vi "COP Transport Layer.vi"() -> ()   [LabVIEW 2011]
uses:
  Support Files/JUDP Read Queue Element.ctl
  Support Files/Address.ctl
  Support Files/JUDP Write Queue Element.ctl
  cRIO/Functional Global Variables/Actions for FG's.ctl
panel:
  out "UDP Write Loop":bool
  out "UDP Read Loop":bool
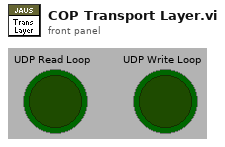
[diagram p1: front panel]
types:
  T1 = typedef "JUDP Write Queue Element.ctl" = cluster{"Encoded JAUS Message":string, "Destination ID":u32}
  T2 = typedef "JUDP Read Queue Element.ctl" = cluster{"Payload":string, "Sender ID":T3, "Command Code":u16}
  T3 = typedef "Address.ctl" = cluster{"Subsystem Id":u16, "Node Id":u8, "Component Id":u8}
  T4 = typedef "UDP Base.ctl" = cluster{"UDP Session":refnum<k16>, "UDP Socket Params":T5}
  T5 = typedef "UDP Socket Params.ctl" = cluster{"Local Port":u16, "Read Timeout":i32, "Write Timeout":i32}
  T6 = typedef "Actions for FG's.ctl" = enum16{"Read", "Write"}
  T7 = cluster{"QueryType":u8, "Type":u16, "COP Identification":string}
  T8 = typedef "UDP Network Location.ctl" = cluster{"IP Address":string, "Port":u16}
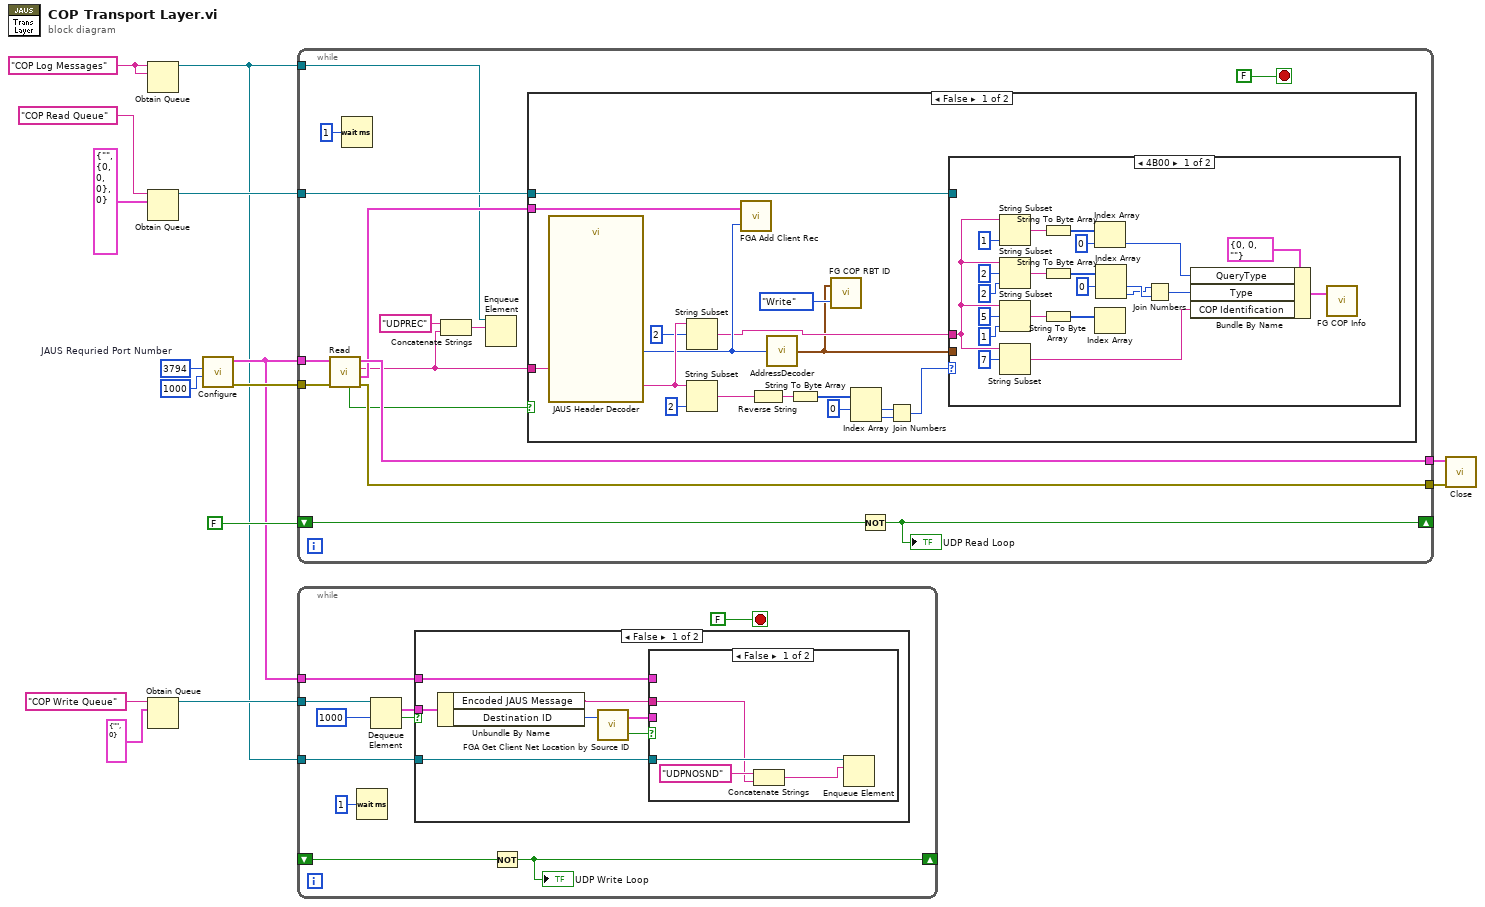
[diagram p0: block diagram]
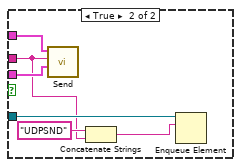
[diagram p2: hidden frame]
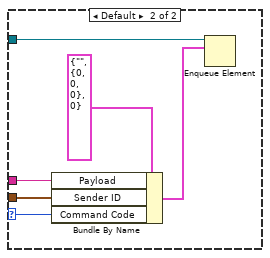
[diagram p4: hidden frame]
diagram:
  w2 = "COP Log Messages" ("name (unnamed)")
  w11 = u16 3794  # JAUS Requried Port Number
  n1 = Obtain Queue(name (unnamed)=w2, element data type=w2) -> (queue out=w1:refnum<queue>)  [unwired: 3 in, 2 out]
  n2 = Obtain Queue(name (unnamed)="COP Read Queue", element data type=T2 {"Payload"="", "Sender ID"={"Subsystem Id"=0, "Node Id"=0, "Component Id"=0}, "Command Code"=0} ("Receive FSM Queue Element")) -> (queue out=w13:refnum<queue>)  [unwired: 3 in, 2 out]
  n3 = Obtain Queue(name (unnamed)="COP Write Queue", element data type=T1 {"Encoded JAUS Message"="", "Destination ID"=0} ("Cluster")) -> (queue out=w6:refnum<queue>)  [unwired: 3 in, 2 out]
  n4 = call "Configure.vi"("Read Timeout"=1000, "Local Port"=w11) -> ("error out"=w12:errorcluster, "UDP Base out"=w3:T4)  [unwired: 8 in]
  n5 = while {
    tunnel: w13 -> [w30]
    tunnel: w3 -> [w28]
    tunnel: w12 -> [w29]
    tunnel: [w27] -> w9
    tunnel: [w26] -> w8
    shift-right: [w24] -> _
    shift-left: FALSE ("stop") -> [w25]
    tunnel: w1 -> [w19]
    stop <- FALSE stop-if-true
    n6 = call "Read.vi"("error in (no error)"=w29, "UDP Base in"=w28) -> ("error out"=w26:errorcluster, "Network Location"=w22:T8, "Receive Data"=w16:string, "UDP Base out"=w27:T4, "Timeout"=w23:bool)  [unwired: 4 in, 1 out]
    n7 = Wait (ms)(milliseconds to wait=u32 1) -> ()  [unwired: 1 out]
    n8 = Concatenate Strings("UDPREC" ("string"), w16) -> (w18:string)
    n9 = Enqueue Element(queue=w19, element=w18) -> ()  [unwired: 2 in, 3 out]
    n10 = case shown="False" w23 {
      tunnel: w30 -> [w36 _]
      tunnel: w16 -> [w38 _]
      tunnel: w22 -> [w37 _]
      frame False {
        n11 = call "JAUS Header Decoder.vi"("Encoded JAUS Message"=w38) -> ("Source ID (80-95)"=w35:u32, "Payload"=w40:string)  [unwired: 13 in, 12 out]
        n12 = String Subset(string=w40, offset (0)=2) -> (substring=w34:string)  [unwired: 1 in]
        n13 = String Subset(string=w40, length (rest)=2 ("length (rest)")) -> (substring=w41:string)  [unwired: 1 in]
        n14 = call "FGA Add Client Rec.vi"("ID"=w35, "Network Location"=w37) -> ()  [unwired: 1 in, 1 out]
        n15 = Reverse String(1:w41) -> (0:w43:string)
        n16 = call "AddressDecoder.vi"("Address"=w35) -> ("Address Cluster"=w31:T3)
        n17 = String To Byte Array(string=w43) -> (unsigned byte array=w47:u8[])
        n18 = call "FG COP RBT ID.vi"("FG Action (Read)"=Actions_for_FG's."Write", "RBT ID in"=w31) -> ()  [unwired: 1 out]
        n19 = Index Array(array=w47, index #1=0 ("index")) -> (element #1=w45:u8, element #2=w44:u8)  [unwired: 1 in]
        n20 = Join Numbers(hi=w45, lo=w44) -> ((hi.lo)=w33:u16)
        n21 = case shown="4B00" w33 {
          selector: w33 -> [_ w70]
          tunnel: w36 -> [_ w75]
          tunnel: w31 -> [_ w74]
          tunnel: w34 -> [w59 w73]
          frame 19200 {
            n22 = String Subset(string=w59, length (rest)=1 ("length (rest)")) -> (substring=w69:string)  [unwired: 1 in]
            n23 = String Subset(string=w59, offset (0)=2, length (rest)=2 ("length (rest)")) -> (substring=w68:string)
            n24 = String Subset(string=w59, offset (0)=5, length (rest)=1 ("length (rest)")) -> (substring=w60:string)
            n25 = String Subset(string=w59, offset (0)=7) -> (substring=w56:string)  [unwired: 1 in]
            n26 = String To Byte Array(string=w69) -> (unsigned byte array=w55:u8[])
            n27 = String To Byte Array(string=w68) -> (unsigned byte array=w51:u8[])
            n28 = String To Byte Array(string=w60) -> (unsigned byte array=w63:u8[])
            n29 = Index Array(array=w55, index=0) -> (element=w53:u8)
            n30 = Index Array(array=w63) -> ()  [unwired: 1 in, 1 out]
            n31 = Index Array(array=w51, index #1=0 ("index")) -> (element #1=w50:u8, element #2=w49:u8)  [unwired: 1 in]
            n32 = Join Numbers(hi=w49, lo=w50) -> ((hi.lo)=w48:u16)
            n33 = Bundle By Name(cluster=T7 {"QueryType"=0, "Type"=0, "COP Identification"=""} ("COP Info in"), "QueryType"=w53, "Type"=w48, "COP Identification"=w56) -> (w57:T7)
            n34 = call "FG COP Info.vi"("COP Info in"=w57) -> ()  [unwired: 1 in, 1 out]
          }
          frame Default {
            n35 = Bundle By Name(cluster=T2 {"Payload"="", "Sender ID"={"Subsystem Id"=0, "Node Id"=0, "Component Id"=0}, "Command Code"=0} ("element"), "Payload"=w73, "Sender ID"=w74, "Command Code"=w70) -> (w71:T2)
            n36 = Enqueue Element(queue=w75, element=w71) -> ()  [unwired: 2 in, 3 out]
          }
        }
      }
      frame True {
      }
    }
    n37 = Not(x=w25) -> (.not. x?=w24:bool)
    "UDP Read Loop" <- w24
  }
  n38 = while {
    shift-right: [w84] -> _
    shift-left: _ -> [w85]
    tunnel: w6 -> [w83]
    tunnel: w3 -> [w80]
    tunnel: w1 -> [w76]
    stop <- FALSE stop-if-true
    n39 = Wait (ms)(milliseconds to wait=u32 1) -> ()  [unwired: 1 out]
    n40 = Dequeue Element(queue=w83, timeout in ms (-1)=1000) -> (element=w81:T1, timed out?=w82:bool)  [unwired: 1 in, 2 out]
    n41 = case shown="False" w82 {
      tunnel: w81 -> [w91 _]
      tunnel: w80 -> [w92 _]
      tunnel: w76 -> [w86 _]
      frame False {
        n42 = Unbundle By Name(w91) -> ("Encoded JAUS Message"=w90:string, "Destination ID"=w89:u32)
        n43 = call "FGA Get Client Net Location by Source ID.vi"("ID"=w89) -> ("Record Exists?"=w88:bool, "Network Location"=w87:T8)  [unwired: 1 in]
        n44 = case shown="False" w88 {
          tunnel: w92 -> [_ w102]
          tunnel: w90 -> [w93 w98]
          tunnel: w87 -> [_ w101]
          tunnel: w86 -> [w94 w100]
          frame False {
            n45 = Concatenate Strings("UDPNOSND" ("string"), w93) -> (w95:string)
            n46 = Enqueue Element(queue=w94, element=w95) -> ()  [unwired: 2 in, 3 out]
          }
          frame True {
            n47 = call "Send.vi"("Destination Location"=w101, "Send Data"=w98, "UDP Base in"=w102) -> ()  [unwired: 6 in, 3 out]
            n48 = Concatenate Strings("UDPSND" ("string"), w98) -> (w97:string)
            n49 = Enqueue Element(queue=w100, element=w97) -> ()  [unwired: 2 in, 3 out]
          }
        }
      }
      frame True {
      }
    }
    n50 = Not(x=w85) -> (.not. x?=w84:bool)
    "UDP Write Loop" <- w84
  }
  n51 = call "Close.vi"("error in (no error)"=w8, "Cluster of class private data"=w9) -> ()  [unwired: 9 in, 1 out]
